vi "Is an Async Methods Actor.vi"(2 "Class in":refnum<vi>) -> (15 "Class out":refnum<vi>, 16 "Is Async Method Actor?":bool, 18 "Async AF Library FQN":string)   [LabVIEW 2023, in "Add Async Methods Actor.lvlib" / "Live Store.lvclass"]
uses:
  Live Store.lvclass
  Live Store.lvclass/Live Store.ctl
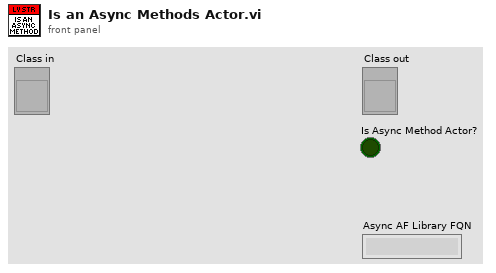
[diagram p1: front panel]
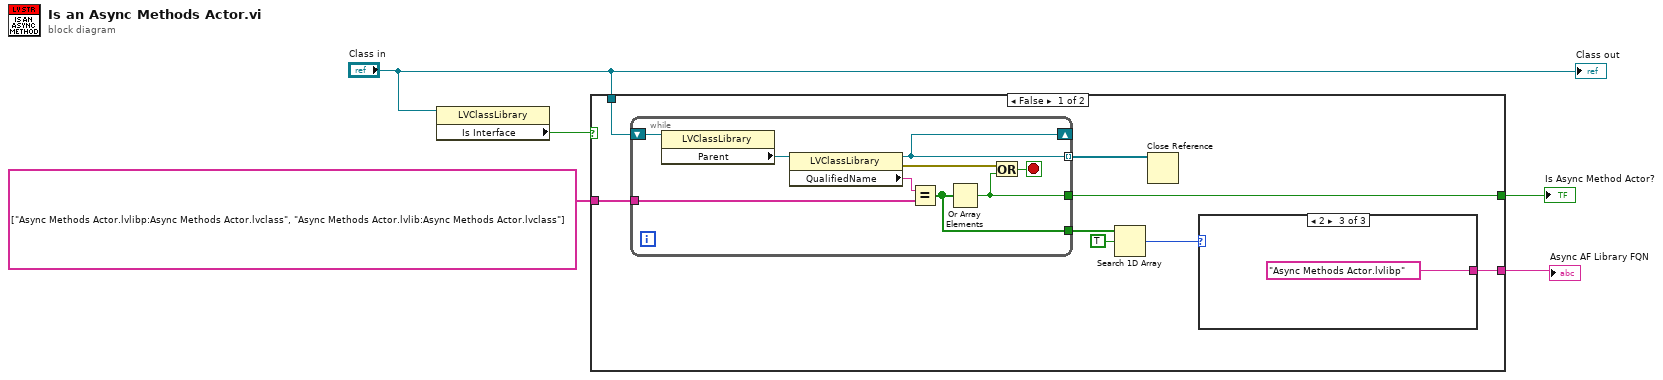
[diagram p0: block diagram]
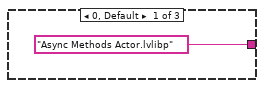
[diagram p2: hidden frame]
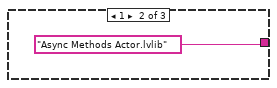
[diagram p3: hidden frame]
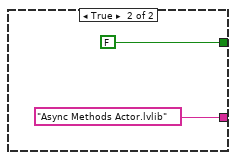
[diagram p4: hidden frame]
diagram:
  n1 = property class="LVClassLibrary"(reference="Class in") -> ("Is Interface"=w3:bool)  [unwired: 1 in, 2 out]
  n2 = case shown="False" w3 {
    tunnel: string[] ["Async Methods Actor.lvlibp:Async Methods Actor.lvclass", "Async Methods Actor.lvlib:Async Methods Actor.lvclass"] -> [w13 _]
    tunnel: "Class in" -> [w8 _]
    tunnel: [w7 FALSE] -> w2
    tunnel: [w6 "Async Methods Actor.lvlib" ("Actor Class")] -> w1
    frame False {
      n3 = while {
        shift-right: [w23] -> _
        shift-left: w8 -> [w25]
        tunnel: [w23] -> w12 mode=indexing
        tunnel: w13 -> [w21]
        tunnel: [w18] -> w7
        tunnel: [w17] -> w11
        stop <- w19 stop-if-true
        n4 = property class="LVClassLibrary"(reference=w25) -> ("Parent"=w24:refnum<vi>)  [unwired: 1 in, 2 out]
        n5 = property class="LVClassLibrary"(reference=w24) -> (reference out=w23:refnum<vi>, error out=w20:errorcluster, "QualifiedName"=w22:string)  [unwired: 1 in]
        n6 = Equal?(x=w22, y=w21) -> (x = y?=w17:bool[])
        n7 = Or Array Elements(Boolean array=w17) -> (logical OR=w18:bool)
        n8 = Or(x=w20, y=w18) -> (x .or. y?=w19:bool)
      }
      n9 = Search 1D Array(1D array=w11, element=TRUE) -> (index of element=w9:i32)  [unwired: 1 in]
      n10 = Close Reference(reference=w12) -> ()  [unwired: 1 in, 1 out]
      n11 = case shown="2" w9 {
        tunnel: ["Async Methods Actor.lvlibp" ("Actor Class") "Async Methods Actor.lvlib" ("Actor Class") "Async Methods Actor.lvlibp" ("Actor Class")] -> w6
        frame 0, Default {
        }
        frame 1 {
        }
        frame 2 {
        }
      }
    }
    frame True {
    }
  }
  "Is Async Method Actor?" <- w2
  "Async AF Library FQN" <- w1
  "Class out" <- "Class in"
